vi "A33ConfigureRamp_py.vi"(8 "error in (no error)":errorcluster, 9 "Ramp symmetry (50%)":dbl=50.0 format="%#_12g", 10 "Channel (1: Channel1)":i32(ring)=1 items=["Channel1"=1, "Channel2"=2]) -> (0 "error out":errorcluster)   [LabVIEW 2022 SP3]
doc: "Selects the waveform shape, frequency, amplitude, offset, and phase for a standard waveform."
uses:
  <vilib>/addons/zeromq/zmq_socket.lvclass
panel:
  out "Standalone":bool
  out "socket out":refnum<class "zmq_socket.lvclass">
  in  "socket in":refnum<class "zmq_socket.lvclass">
  out "resulting string":string
  in  "Instrument":string="AG33600A_Gen1"
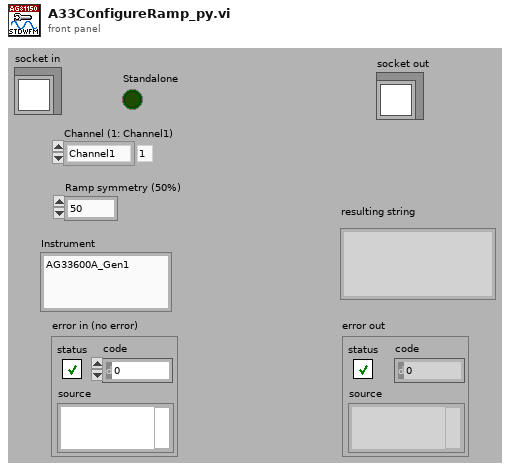
[diagram p1: front panel]
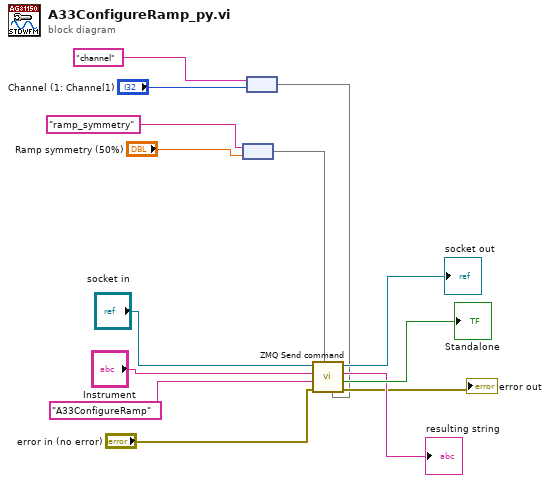
[diagram p0: block diagram]
diagram:
  n1 = node("ramp_symmetry" ("key"), "Ramp symmetry (50%)") -> (w4:map{string, dbl})
  n2 = node("channel" ("key"), "Channel (1: Channel1)") -> (w1:map{string, i32})
  n3 = call "ZMQ Send command.vi"("Int args"=w1, "DBL args"=w4, "error in"="error in (no error)", "Command"="A33ConfigureRamp", "Instrument"="Instrument", "socket in"="socket in") -> ("error out"=→"error out":errorcluster, "Standalone"=→"Standalone":bool, "Recieved message"=→"resulting string":string, "socket out"=→"socket out":refnum<class "zmq_socket.lvclass">)  [unwired: 2 in]
